vi "RotateX.vi"(1 "theta":dbl) -> (0 "rotation matrix":T1)   [LabVIEW 2021]
doc: "Rotate X-axis."
uses:
  <vilib>/Analysis/Matrix/Datatypes/RealMatrix.ctl
  <vilib>/Analysis/Matrix/NI_Matrix.lvlib
panel:
  # "Rotate X-axis."
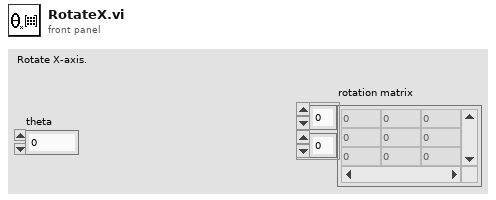
[diagram p1: front panel]
types:
  T1 = typedef "NI_Matrix.lvlib/RealMatrix.ctl" = dbl[][]
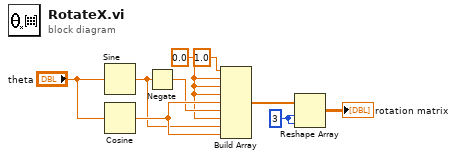
[diagram p0: block diagram]
diagram:
  w1 = 0.0
  w8 = 3 ("number of rows")
  n1 = Sine(x="theta") -> (sin(x)=w2:dbl)
  n2 = Cosine(x="theta") -> (cos(x)=w4:dbl)
  n3 = Negate(x=w2) -> (-x=w3:dbl)
  n4 = Build Array(1.0, w1, w1, w1, w4, w3, w1, w2, w4) -> (w9:dbl[])
  n5 = Reshape Array(w9, w8, w8) -> (→"rotation matrix":dbl[][])
